vi "test_SessionAlreadyInitialized_InitializeSessions_ReturnsError.vi"(8 "error in":errorcluster) -> (0 "error out":errorcluster, 2 "result":string, 3 "pass":bool)   [LabVIEW 2020, in "MeasurementServerTests.lvlib"]
uses:
  MeasurementServerTests.lvlib
  Helpers/Fake Session Factory/Fake Session Factory.lvclass
  da6ffb6f-c1c9-4957-84dd-e9228483c454.vi
  Runtime/Measurements/Helpers/Error Strings Global Internal.vi
  ffc64c76-1568-41a3-8328-b9126ac9a28d.vi
  Runtime/APIs/Session Management V1/Session Reservation/Initialize and Close Session Behavior.ctl
  Runtime/APIs/Session Management V1/Session Reservation/Session Reservation.lvclass
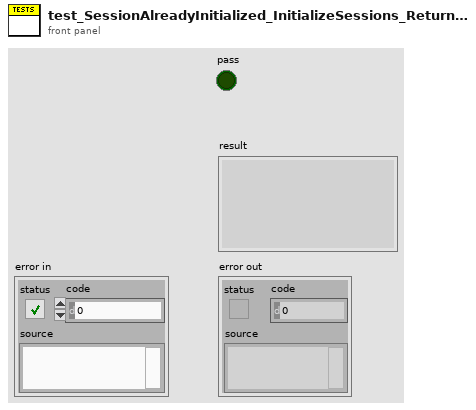
[diagram p1: front panel]
types:
  T1 = typedef "Plug-In SDK Session Management V1 API.lvlib/Session Reservation.lvclass/Initialize and Close Session Behavior.ctl" = enum16{"Auto", "Initialize and Close", "Attach and Detach", "Initialize and Detach", "Attach and Close"}
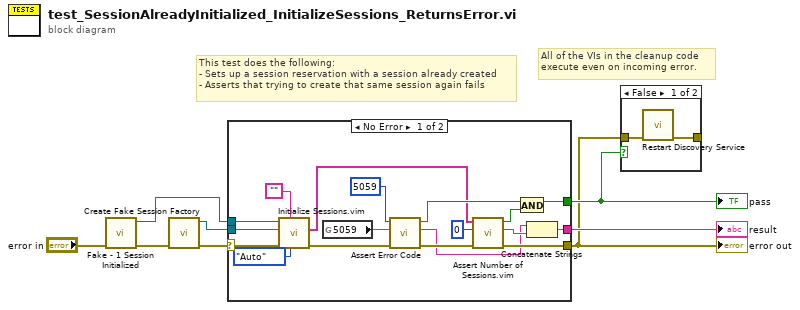
[diagram p0: block diagram]
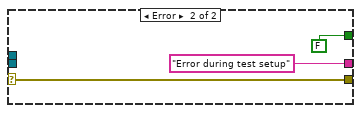
[diagram p2: hidden frame]
diagram:
  # "All of the VIs in the cleanup code\nexecute even on incoming error."
  # "This test does the following:\n- Sets up a session reservation with a session already created\n- Asserts that trying to create that same session again fails"
  n1 = call "Fake - 1 Session Initialized.vi"("error in"="error in") -> ("error out"=w2:errorcluster, "session reservation out"=w1:refnum<class "Session Reservation.lvclass">)  [unwired: 9 in]
  n2 = call "Create Fake Session Factory.vi"("error in"=w2) -> ("error out"=w5:errorcluster, "fake session factory out"=w4:refnum<class "Fake Session Factory.lvclass">)  [unwired: 9 in]
  n3 = case shown="No Error" w5 {
    selector: w5 -> [w24 w27]
    tunnel: [w15 w27] -> w6
    tunnel: [w14 FALSE] -> w7
    tunnel: [w12 "Error during test setup" ("f")] -> w8
    tunnel: w4 -> [w26 _]
    tunnel: w1 -> [w25 _]
    frame No Error {
      n4 = call "Initialize Sessions.vim"("initialize and close session behavior"=Initialize_and_Close_Session_Behavior."Auto", "session type"="", "error in"=w24, "session factory"=w26, "session reservation in"=w25) -> ("error out"=w23:errorcluster, "sessions"=w18:string[])  [unwired: 3 in, 2 out]
      n5 = global read "Error Strings Global Internal.vi" "5059"() -> (w19:string)
      n6 = call "Assert Error Code.vi"("error in"=w23, "expected error description"=w19, "expected error code"=5059) -> ("error out"=w16:errorcluster, "details"=w10:string, "error code match?"=w22:bool)  [unwired: 6 in]
      n7 = call "Assert Number of Sessions.vim"("error in"=w16, "expected number of sessions"=0, "sessions"=w18) -> ("error out"=w15:errorcluster, "result"=w11:string, "pass"=w13:bool)  [unwired: 6 in]
      n8 = And(x=w22, y=w13) -> (x .and. y?=w14:bool)
      n9 = Concatenate Strings(w10, w11) -> (w12:string)
    }
    frame Error {
    }
  }
  "error out" <- w6
  "pass" <- w7
  "result" <- w8
  n10 = case shown="False" w7 {
    tunnel: w6 -> [w31 _]
    tunnel: [w30 _] -> _
    frame False {
      n11 = call "Restart Discovery Service.vi"("error in"=w31) -> ("error out"=w30:errorcluster)  [unwired: 10 in]
    }
    frame True {
    }
  }
